vi "Start.vi"(8 "error in (no error)":errorcluster, 11 "Scope PXI in":refnum<class "Scope PXI.lvclass">) -> (0 "error out":errorcluster, 3 "Scope PXI out":refnum<class "Scope PXI.lvclass">)   [LabVIEW 2023, in "Scope PXI.lvlib" / "Scope PXI.lvclass"]
uses:
  Scope PXI.lvclass
  Scope PXI.lvclass/Scope PXI.ctl
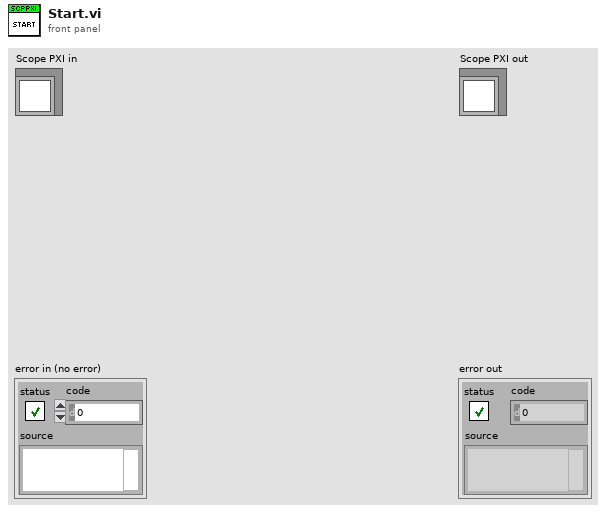
[diagram p1: front panel]
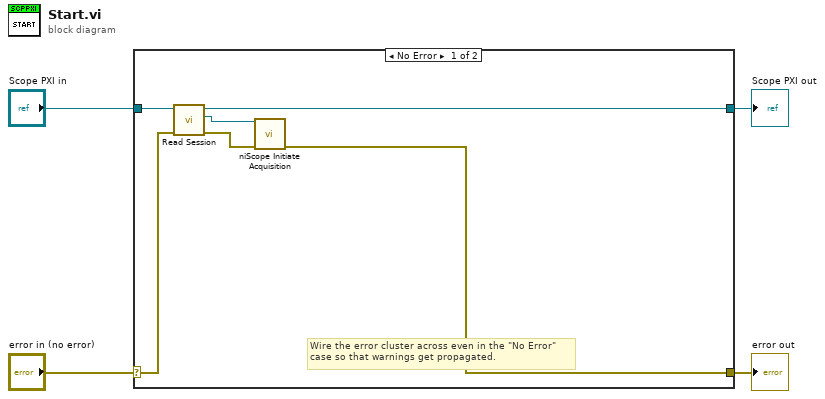
[diagram p0: block diagram]
diagram:
  n1 = case shown="No Error" "error in (no error)" {
    selector: "error in (no error)" -> [w10 w12]
    tunnel: [w6 w12] -> w3
    tunnel: [w7 w11] -> w1
    tunnel: "Scope PXI in" -> [w8 w11]
    frame No Error {
      # "Wire the error cluster across even in the \"No Error\"\ncase so that warnings get propagated."
      n2 = call "Read Session.vi"("error in (no error)"=w10, "Scope PXI in"=w8) -> ("error out"=w9:errorcluster, "session"=w5:refnum<k15>, "Scope PXI out"=w7:refnum<class "Scope PXI.lvclass">)  [unwired: 7 in]
      n3 = call <instrlib>:"niScope Initiate Acquisition.vi"("instrument handle"=w5, "error in"=w9) -> ("error out"=w6:errorcluster)  [unwired: 12 in, 1 out]
    }
    frame Error {
    }
  }
  "error out" <- w3
  "Scope PXI out" <- w1
